vi "get supported channel classifications.vi"(8 "error in":errorcluster, 11 "module configuration in":refnum<class "TBM module configuration.lvclass">) -> (0 "error out":errorcluster, 2 "supported types":T1[](array[typedef]), 3 "module configuration out":refnum<class "TBM module configuration.lvclass">)   [LabVIEW 2013, in "TBM module configuration.lvclass"]
doc: "Provides an interface for determining the channel types supported by a given configuration/runtime class pairing. This should be overridden by a child class in order to allow for improved validation of a given configuration."
uses:
  TBM module configuration.lvclass
  channel/channel classification.ctl
  channel/TBM channel.lvclass
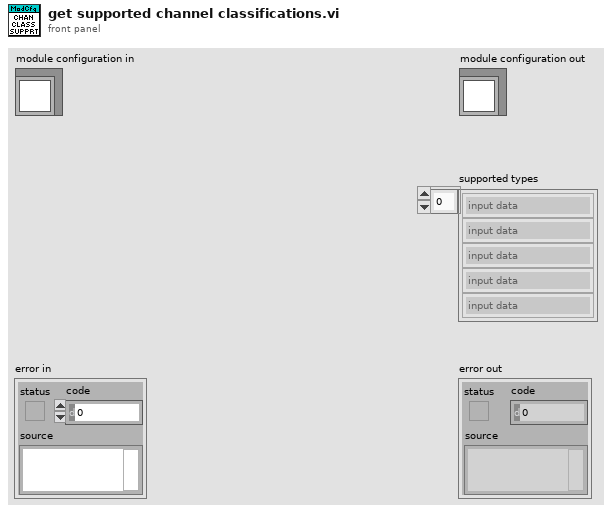
[diagram p1: front panel]
types:
  T1 = typedef "TBM channel.lvclass/channel classification.ctl" = enum16{"input data", "output data", "processing parameter", "processing result"}
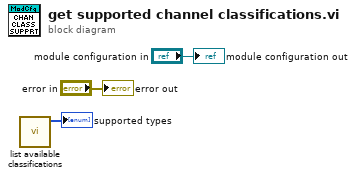
[diagram p0: block diagram]
diagram:
  n1 = call "list available classifications.vi"() -> ("supported types"=→"supported types":T1[])  [unwired: 11 in]
  "error out" <- "error in"
  "module configuration out" <- "module configuration in"
